vi "Stop Receiving.vi"(8 "error in (no error)":errorcluster, 11 "UDP Data Receiver in":refnum<class "UDP Data Receiver.lvclass">) -> (0 "error out":errorcluster, 3 "UDP Data Receiver out":refnum<class "UDP Data Receiver.lvclass">)   [LabVIEW 2022 SP3, in "UDP Data Receiver.lvlib" / "UDP Data Receiver.lvclass"]
uses:
  UDP Data Receiver.lvclass
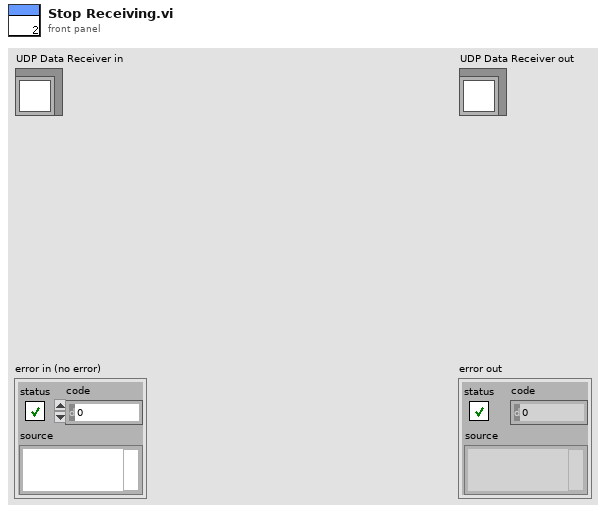
[diagram p1: front panel]
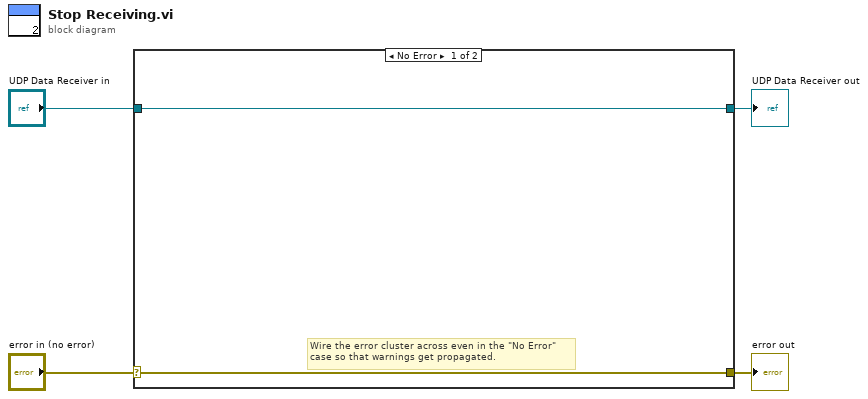
[diagram p0: block diagram]
diagram:
  n1 = case shown="No Error" "error in (no error)" {
    selector: "error in (no error)" -> [w5 w8]
    tunnel: [w5 w8] -> w3
    tunnel: [w6 w7] -> w1
    tunnel: "UDP Data Receiver in" -> [w6 w7]
    frame No Error {
      # "Wire the error cluster across even in the \"No Error\"\ncase so that warnings get propagated."
    }
    frame Error {
    }
  }
  "error out" <- w3
  "UDP Data Receiver out" <- w1
